vi "Start.vi"(8 "error in (no error)":errorcluster, 11 "Motor-GWInstek in":refnum<class "Motor-GWInstek.lvclass">) -> (0 "error out":errorcluster, 3 "Motor-GWInstek out":refnum<class "Motor-GWInstek.lvclass">)   [LabVIEW 2013, in "PowderDeposition.lvlib" / "Motor-GWInstek.lvclass"]
uses:
  Motor-GWInstek.lvclass
  Motor-GWInstek.lvclass/Motor-GWInstek.ctl
  Read Channel.vi
  <instrlib>/GPD-2303/GPD-2303.lvlib
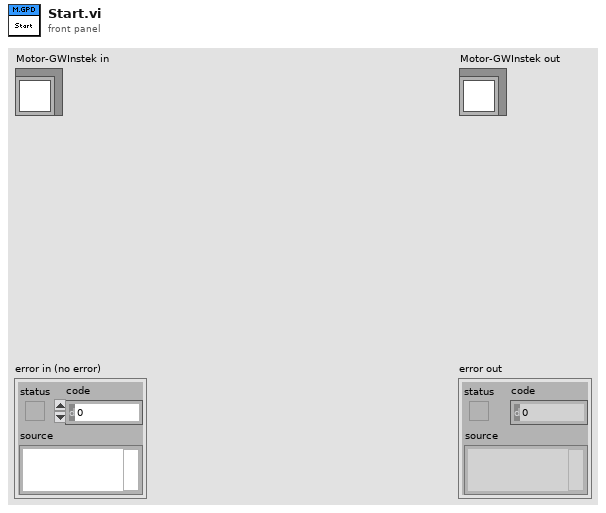
[diagram p1: front panel]
types:
  T1 = typedef "PowderDeposition.lvlib/Motor.lvclass/Action-settings.ctl" = cluster{"Speed":dbl, "Acceleration":dbl, "Direction":enum16{"Clockwise", "Counter-clockwise"}}
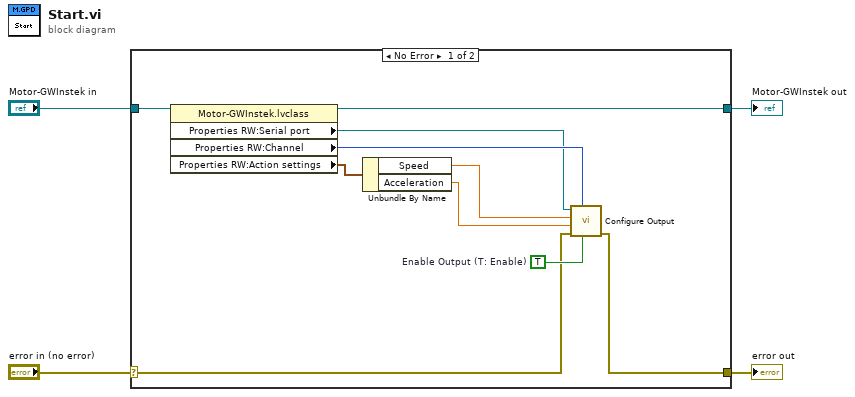
[diagram p0: block diagram]
diagram:
  n1 = case shown="No Error" "error in (no error)" {
    selector: "error in (no error)" -> [w5 w16]
    tunnel: [w13 w16] -> w3
    tunnel: [w11 w15] -> w1
    tunnel: "Motor-GWInstek in" -> [w12 w15]
    frame No Error {
      w14 = TRUE  # Enable Output (T: Enable)
      n2 = property class="Motor-GWInstek.lvclass"(reference=w12) -> (reference out=w11:refnum<class "Motor-GWInstek.lvclass">, "Properties RW:Serial port"=w9:refnum<visa-resource-name>, "Properties RW:Channel"=w10:i32, "Properties RW:Action settings"=w8:T1)  [unwired: 1 in, 1 out]
      n3 = Unbundle By Name(w8) -> ("Speed"=w7:dbl, "Acceleration"=w6:dbl)
      n4 = call <instrlib>:"Configure Output.vi"("Enable Output (T: Enable)"=w14, "Channel (1: Channel 1)"=w10, "error in (no error)"=w5, "Current Level (0.0 V)"=w6, "Voltage Level (0.0 V)"=w7, "VISA resource name"=w9) -> ("error out"=w13:errorcluster)  [unwired: 4 in, 1 out]
    }
    frame Error {
    }
  }
  "error out" <- w3
  "Motor-GWInstek out" <- w1
